vi "Load Picture.vi"(8 "error in (no error)":errorcluster, 11 "Picture Config":T1) -> (0 "error out":errorcluster, 3 "Picture from File":picture)   [LabVIEW 2011]
uses:
  Picture Configuration.ctl
  <vilib>/picture/picture.llb/imagedata.ctl
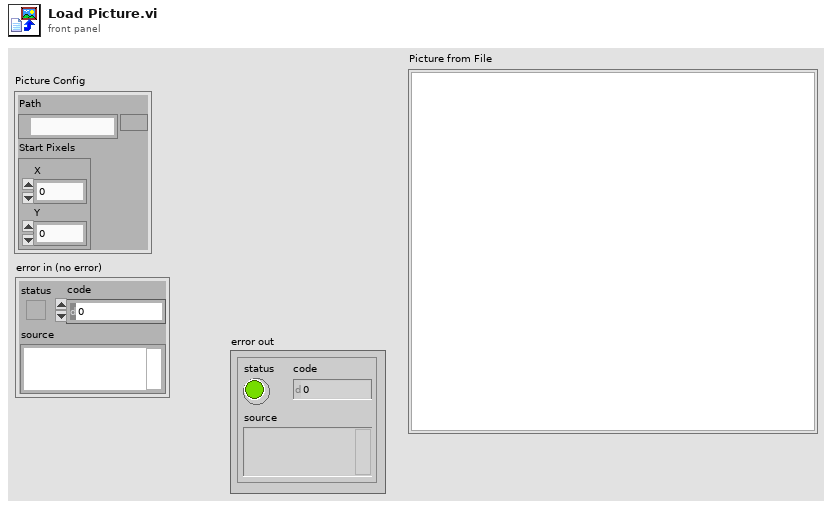
[diagram p1: front panel]
types:
  T1 = typedef "Picture Configuration.ctl" = cluster{"Path":path, "Start Pixels":cluster{"X":i32, "Y":i32}}
  T2 = cluster{"left":i16, "top":i16, "right":i16, "bottom":i16}
  T3 = typedef "imagedata.ctl" = cluster{"image type":i32, "image depth":i32, "image":u8[], "mask":u8[], "colors":u32[], "Rectangle":cluster{"left":i16, "top":i16, "right":i16, "bottom":i16}}
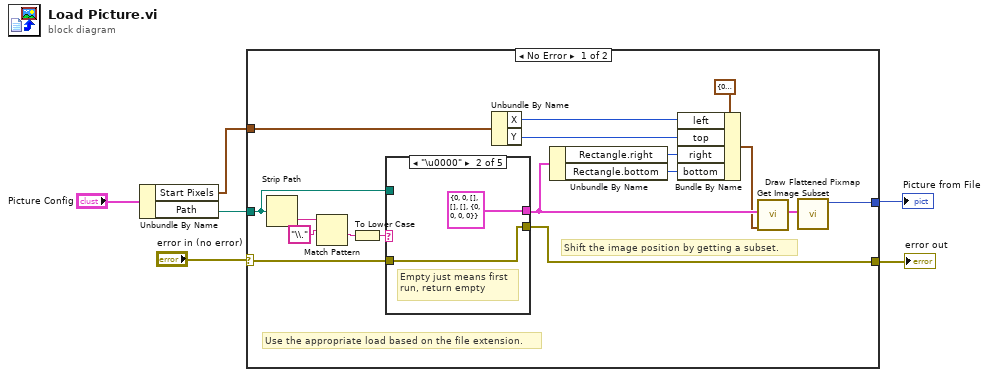
[diagram p0: block diagram]
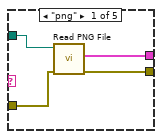
[diagram p2: hidden frame]
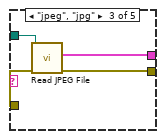
[diagram p3: hidden frame]
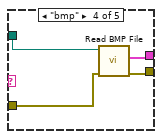
[diagram p4: hidden frame]
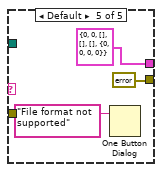
[diagram p5: hidden frame]
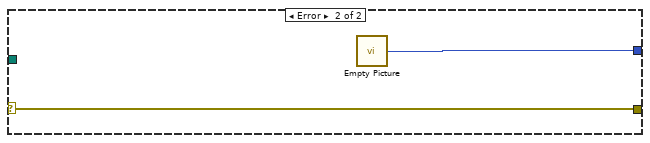
[diagram p6: hidden frame]
diagram:
  n1 = Unbundle By Name("Picture Config") -> ("Start Pixels"=w1:cluster{"X":i32, "Y":i32}, "Path"=w2:path)
  n2 = case shown="No Error" "error in (no error)" {
    selector: "error in (no error)" -> [w18 w42]
    tunnel: w2 -> [w17 _]
    tunnel: [w20 w41] -> w6
    tunnel: [w19 w42] -> w5
    tunnel: w1 -> [w15 _]
    frame No Error {
      # "Shift the image position by getting a subset."
      # "Use the appropriate load based on the file extension."
      n3 = Strip Path(path=w17) -> (name=w23:string)  [unwired: 1 out]
      n4 = Match Pattern(string=w23, regular expression="\\.") -> (after substring=w21:string)  [unwired: 1 in, 3 out]
      n5 = To Lower Case(string=w21) -> (all lower case string=w16:string)
      n6 = case shown="\"\"" w16 {
        tunnel: w17 -> [w27 _ w33 w35 _]
        tunnel: [w26 w28 w31 w37 errorcluster {"status"=FALSE, "code"=0, "source"=""} ("error out")] -> w19
        tunnel: [w25 T3 {"image type"=0, "image depth"=0, "image"=[], "mask"=[], "colors"=[], "Rectangle"={"left"=0, "top"=0, "right"=0, "bottom"=0}} ("image data") w32 w36 T3 {"image type"=0, "image depth"=0, "image"=[], "mask"=[], "colors"=[], "Rectangle"={"left"=0, "top"=0, "right"=0, "bottom"=0}} ("image data")] -> w13
        tunnel: w18 -> [w24 w28 w30 w34 _]
        frame "png" {
          n7 = call <vilib>:"Read PNG File.vi"("error in (no error)"=w24, "path to PNG file"=w27) -> ("error out"=w26:errorcluster, "image data"=w25:T3)  [unwired: 7 in, 1 out]
        }
        frame "\u0000" {
          # "Empty just means first\nrun, return empty"
        }
        frame "jpeg", "jpg" {
          n8 = call <vilib>:"Read JPEG File.vi"("error in (no error)"=w30, "path to JPEG file"=w33) -> ("error out"=w31:errorcluster, "image data"=w32:T3)  [unwired: 7 in, 1 out]
        }
        frame "bmp" {
          n9 = call <vilib>:"Read BMP File.vi"("error in (no error)"=w34, "path to BMP file"=w35) -> ("error out"=w37:errorcluster, "image data"=w36:T3)  [unwired: 7 in, 1 out]
        }
        frame Default {
          n10 = One Button Dialog(message="File format not supported") -> ()  [unwired: 1 in, 1 out]
        }
      }
      n11 = Unbundle By Name(w15) -> ("X"=w11:i32, "Y"=w10:i32)
      n12 = Unbundle By Name(w13) -> ("Rectangle.right"=w9:i16, "Rectangle.bottom"=w8:i16)
      n13 = Bundle By Name(cluster=T2 {"left"=0, "top"=0, "right"=0, "bottom"=0} ("subset rect"), "left"=w11, "top"=w10, "right"=w9, "bottom"=w8) -> (w7:T2)
      n14 = call <vilib>:"Get Image Subset.vi"("subset rect"=w7, "image data"=w13) -> ("image subset"=w14:T3)  [unwired: 4 in, 1 out]
      n15 = call <vilib>:"Draw Flattened Pixmap.vi"("image data"=w14) -> ("new picture"=w20:picture)  [unwired: 8 in]
    }
    frame Error {
      n16 = call "Empty Picture"() -> ("empty picture"=w41:picture)
    }
  }
  "Picture from File" <- w6
  "error out" <- w5
